vi "Scan Engine-Single Frame.vi"(8 "Error in":errorcluster, 10 "Scan Status in":T1) -> (0 "Error Out":errorcluster, 2 "Buffer":u16[](array[numeric]), 3 "FFT Buffer":sgl[](array[numeric]))   [LabVIEW 2018]
uses:
  Controls/scan status.ctl
  Controls/FGV Actions.ctl
  Hardware Mfg/AlazarTech SDK/Controls/Alazar Engine Actions.ctl
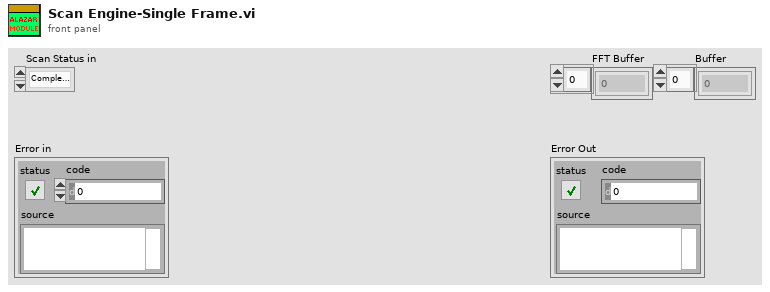
[diagram p1: front panel]
types:
  T1 = typedef "scan status.ctl" = enum16{"Complete Scan(ThorOCT)", "Complete Scan(PSOCT)", "Start(ThorOCT Spatial)", "Start(ThorOCT Spectral)", "Start(GPU FFT)", "Start(Alazar FFT)", "Scan(ThorOCT Spatial)", "Scan(ThorOCT Spectral)", "Scan(GPU FFT)", "Scan(Alazar FFT)", "Finish Scan(ThorOCT)", "Finish Scan(PSOCT)", "Scan(simulate)", "Start(ROI)"}
  T2 = typedef "FGV Actions.ctl" = enum16{"Init", "Set", "Get", "Clear"}
  T3 = typedef "System Parameters.ctl" = cluster{"Optical Parameters":T4, "Vibratome":T5, "Table Stages":T7, "Imaging Parameter":T10, "Galvo HW Parameters":cluster{"Analog Out Channel":tag, "Min Voltage":dbl, "Max Voltage":dbl, "Pixel Clock Source":tag, "Sample Rate":dbl, "Line Clock Out Ch":tag, "2P ready check":tag}, "Alazar parameters":T12, "Mosaic Paramter":cluster{"X Axis":cluster{"Start [mm]":dbl, "Steps [pts]":dbl, "End [mm]":dbl}, "Y Axis":cluster{"Start [mm]":dbl, "Steps [pts]":dbl, "End [mm]":dbl}, "Scan Pattern":enum16{"Uni-directional", "Bi-Directional", "Spiral Out", "Spiral In"}, "Overlap Options":cluster{"Overlap Type":enum16{"No Overlap", "X Only", "Y Only", "X and Y"}, "Percent Overlap":u8, "Justify":enum16{"Start", "Center", "End"}}}, "Manual Controls":T19, "Z stage setting":T23, "Attenuator":T24}
  T4 = typedef "Optical Parameters.ctl" = cluster{"Obj. Focal Length [mm]":dbl, "Scan Lens EFL[mm]":dbl, "Tube Lens EFL[mm]":dbl, "Galvo V Range (+/-)":dbl, "Galvo Max Half Angle [Deg]":dbl, "Max Galvo Range[%]":dbl}
  T5 = typedef "Vibratome Parameters.ctl" = cluster{"Pre Cut Dwell [s]":dbl, "Blade Frequency [RPM]":u16, "Slice Speed [mm/s]":dbl, "Post Cut Dwell [s]":dbl, "Ramp Time [s]":dbl, "Start X [mm]":dbl, "Start Y [mm]":dbl, "Slice Length [mm]":dbl, "Slice Axis":enum16{"X Axis", "Y Axis", "Z Axis"}, "Controller VISA Ref":refnum<visa-resource-name>, "Blade Frequency [Hz]":u16, "Analog Out Channel":tag, "Pixel Clock Source":tag, "Vib version":T6}
  T6 = typedef "vibratome.ctl" = enum16{"Vibratome1", "Vibratome3"}
  T7 = typedef "Translation Stage Parameters.ctl" = cluster{"X Stage":T8, "Y Stage":T8, "Z Stage":T8, "Attenuator":T8}
  T8 = typedef "Translation Stage Cluster.ctl" = cluster{"Position":dbl, "Is.Enabled?":bool, "Is.Connected?":bool, "Device SN":string, "AccelerationMaximum":dbl, "VelocityMaximum":dbl, "Acceleration":dbl, "Velocity":dbl, "waitTimeout (ms)":i32, "Model":T9, "Is.Homed?":bool, "MOVE":bool}
  T9 = typedef "Translation Stage Types.ctl" = enum16{"None", "Thorlabs LTS", "Thorlabs MLJ"}
  T10 = typedef "Imaging Parameters.ctl" = cluster{"Raster Scan Direction":T11, "Pixel Dwell Time [Clock Cycles]":u16, "Flyback Time [Clock Cycles]":u16, "XY Center [um]":cluster{"X":dbl, "Y":dbl}, "Pixel Step Size [um] X":dbl, "XY Image Size":enum16{"32 x 32", "64 x 64", "128 x 128", "256 x 256", "512 x 512", "1024 x 1024", "2048 x 2048"}, "Custom":bool, "Custom Size":cluster{"X":u16, "Y":u16}, "Line Averages":u16, "Pixel Step Size [um] Y":dbl}
  T11 = typedef "Scan Direction.ctl" = enum16{"Uni Directional", "Bi Directional", "None"}
  T12 = typedef "Alazar parameters.ctl" = cluster{"Trigger Settings":cluster{"General Trigger Settings":T13, "Trigger Engine 1":T14, "Trigger Engine 2":T14}, "Device ID":T15, "Ch A Input Control":T16, "Ch B Input Control":T16, "Acq Settings":T17, "Capture Clock":T18}
  T13 = typedef "General Trigger Settings.ctl" = cluster{"Trigger Operation":u32, "Coupling ID":u32, "Range ID":u32, "Delay":u32, "Timeout Ticks":u32, "Mode":u32, "Parameter":u32}
  T14 = typedef "Trigger Engine Controls.ctl" = cluster{"Trigger Engine":u32, "Source":u32, "Slope":u32, "Level":u32}
  T15 = typedef "Alazar Device ID.ctl" = cluster{"System ID":u32, "Board ID":u32}
  T16 = typedef "Channel Input Controls.ctl" = cluster{"Channel":u8, "Coupling":u32, "Range":u32, "Impedance":u32}
  T17 = typedef "Alazar Acquisition Settings.ctl" = cluster{"Record Length":u32, "Offset":u32, "Records Per Buffer":u32, "Records Count (Records/Acq)":u32, "Window Type":u32, "Footer":u32, "Samples per record":u32, "Output Format":u32}
  T18 = typedef "Clock Controls.ctl" = cluster{"Sample Rate":u32, "Decimation":u32, "Source":u32, "Edge":u32}
  T19 = typedef "Manual Controls.ctl" = cluster{"Data Path":path, "Save parameters":T20, "Acquisition mode":T21, "PSOCT Channel":u32, "Save data?":bool, "AIP rotation angle":dbl, "Pause acquisition?":bool, "Outgoing Mail Server (SMTP)":string, "Email":string, "Password":string, "Carrier 1":enum16{"T-Mobile", "AT&T", "Verizon", "Sprint"}, "phone number 1":string, "Subject":string, "Message":string, "Carrier 2":enum16{"T-Mobile", "AT&T", "Verizon", "Sprint"}, "phone number 2":string, "Check boundary?":bool, "Threshold":sgl, "Outputs for GPU FFT":T22, "Slice# init":i32}
  T20 = typedef "FFT parameters.ctl" = cluster{"start pixel":i32, "#pixels to save":i32}
  T21 = typedef "FFT mode.ctl" = enum16{"ThorOCT B line", "ThorOCT Spectral", "ThorOCT FFT", "Alazar B line", "Alazar FFT", "GPU FFT", "Alazar Spectral", "Simulation", "auto adjust focus", "Save all"}
  T22 = typedef "GPU FFT outputs.ctl" = enum16{"Amp + Phase diff", "Amp + Phase", "Amp only"}
  T23 = typedef "Vibratome Param.ctl" = cluster{"first cut height(mm)":dbl, "slice thickness[um]":dbl[], "#repetitions":u16, "image thickness(um)":dbl[], "#cycles per repetition":u16, "First image height(mm)":dbl, "Block?":bool[], "Z0":dbl, "fixed Z0?":bool}
  T24 = typedef "attenuator.ctl" = cluster{"Power after Objective (recalibrate every 6 month)":dbl[]}
  T25 = typedef "Alazar Engine Actions.ctl" = enum16{"Init", "Config Clock", "Config Ch", "Config Trig", "Config Non-FFT Acq.", "Non-FFT Acquire", "start acquire", "Config Acq.", "Acquire", "UnInit"}
  T26 = enum16{"Configure channels", "Write Scan Pattern", "Start Galvo Task", "Is Task Done?", "Stop Galvo", "Uninit", "Init: Calc scan pattern"}
  T27 = cluster{"General Trigger Settings":T13, "Trigger Engine 1":T14, "Trigger Engine 2":T14}
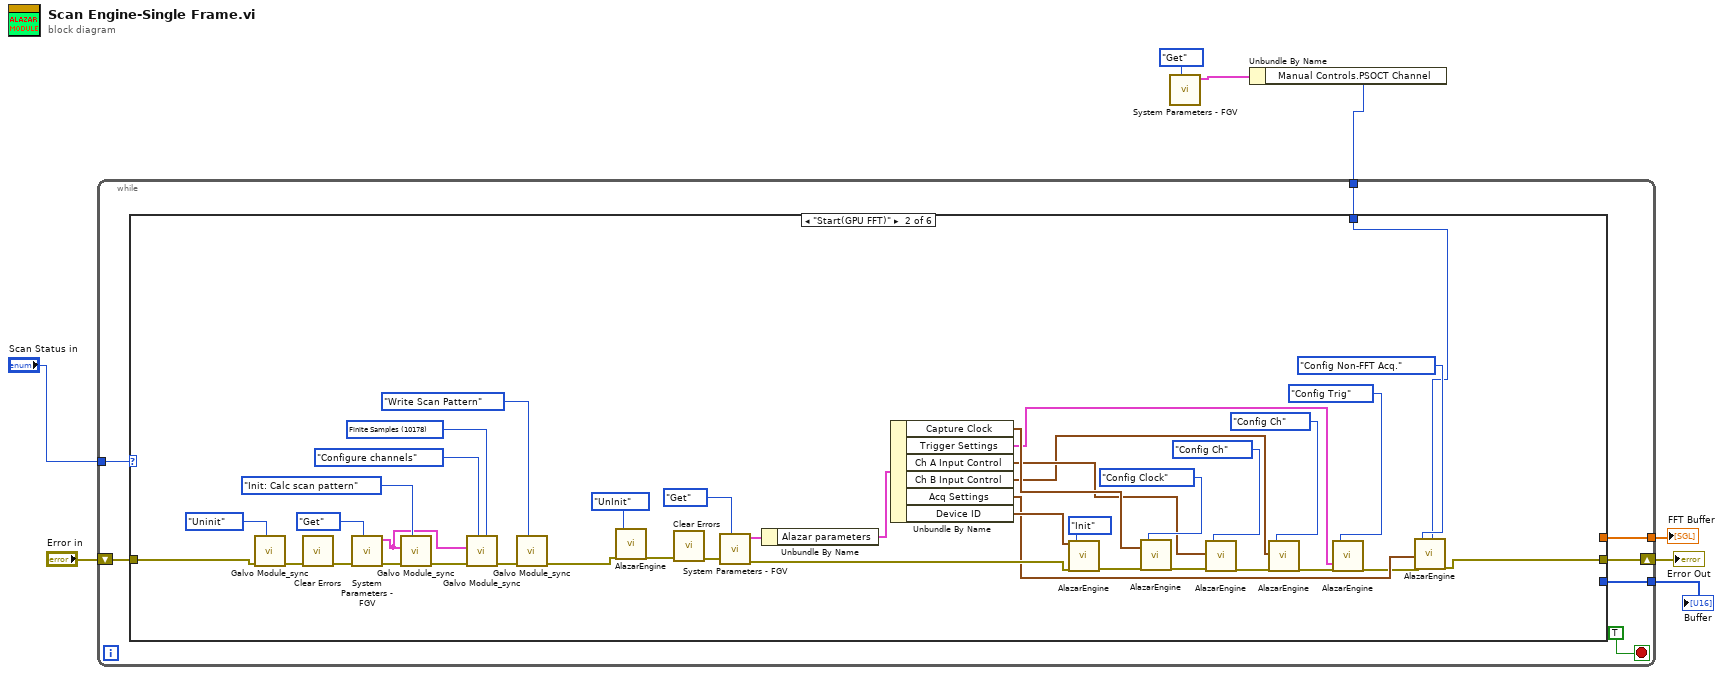
[diagram p0: block diagram]
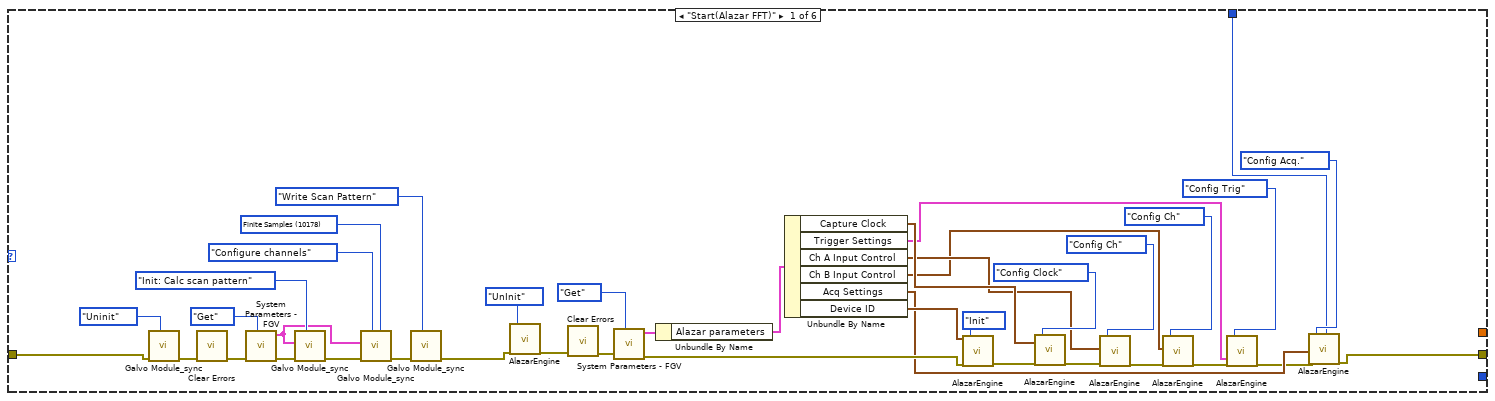
[diagram p2: hidden frame]
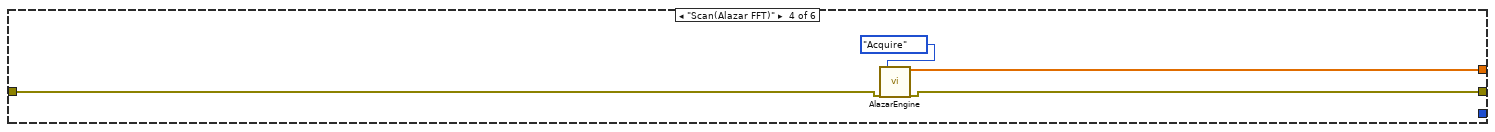
[diagram p4: hidden frame]
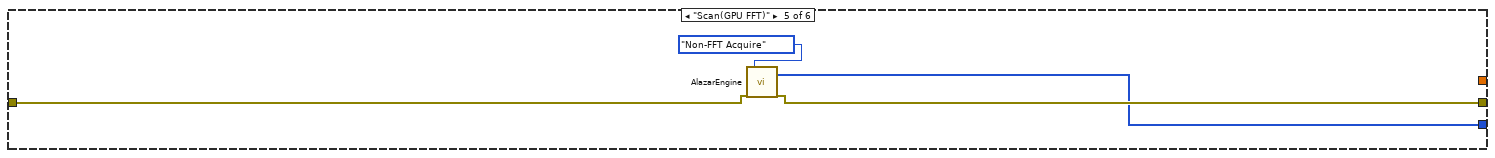
[diagram p5: hidden frame]
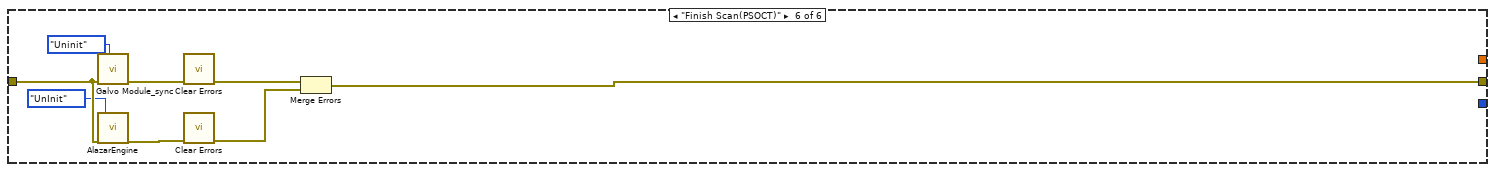
[diagram p6: hidden frame]
diagram:
  n1 = call "System Parameters - FGV.vi"("Actions"=FGV_Actions."Get") -> ("System Parameters [Out]"=w2:T3)  [unwired: 9 in, 1 out]
  n2 = Unbundle By Name(w2) -> ("Manual Controls.PSOCT Channel"=w1:u32)
  n3 = while {
    shift-right: [w14] -> w7
    shift-left: "Error in" -> [w12]
    tunnel: "Scan Status in" -> [w13]
    tunnel: [w11] -> w5
    tunnel: [w10] -> w4
    tunnel: w1 -> [w9]
    stop <- TRUE ("Status In") stop-if-true
    n4 = case shown="\"Start(GPU FFT)\"" w13 {
      tunnel: w12 -> [w44 w59 w96 w99 w103 w109]
      tunnel: [w18 w58 w96 w98 w102 w106] -> w14
      tunnel: [_ _ _ w97 _ _] -> w11
      tunnel: [_ _ _ _ w101 _] -> w10
      tunnel: w9 -> [w17 w57 _ _ _ _]
      frame "Start(Alazar FFT)" {
        w52 = 10178 items=["Finite Samples"=10178, "Continuous Samples"=10123, "Hardware Timed Single Point"=12522] ("sample mode")
        n5 = call "Galvo Module_sync.vi"("Action"=T26."Uninit", "error in (no error)"=w44) -> ("error out"=w47:errorcluster)  [unwired: 8 in, 1 out]
        n6 = call <vilib>:"Clear Errors.vi"("error in (no error)"=w47) -> ("error out"=w45:errorcluster)  [unwired: 5 in, 1 out]
        n7 = call "System Parameters - FGV.vi"("Actions"=FGV_Actions."Get", "Error In"=w45) -> ("Error Out"=w48:errorcluster, "System Parameters [Out]"=w16:T3)  [unwired: 8 in]
        n8 = call "Galvo Module_sync.vi"("Action"=T26."Init: Calc scan pattern", "error in (no error)"=w48, "System Parameters"=w16) -> ("error out"=w54:errorcluster)  [unwired: 7 in, 1 out]
        n9 = call "Galvo Module_sync.vi"("sample mode"=w52, "Action"=T26."Configure channels", "error in (no error)"=w54, "System Parameters"=w16) -> ("error out"=w55:errorcluster)  [unwired: 6 in, 1 out]
        n10 = call "Galvo Module_sync.vi"("Action"=T26."Write Scan Pattern", "error in (no error)"=w55) -> ("error out"=w39:errorcluster)  [unwired: 8 in, 1 out]
        n11 = call "AlazarEngine.vi"("error in (no error)"=w39, "Action"=Alazar_Engine_Actions."UnInit") -> ("error out"=w38:errorcluster)  [unwired: 15 in, 2 out]
        n12 = call <vilib>:"Clear Errors.vi"("error in (no error)"=w38) -> ("error out"=w40:errorcluster)  [unwired: 5 in, 1 out]
        n13 = call "System Parameters - FGV.vi"("Actions"=FGV_Actions."Get", "Error In"=w40) -> ("Error Out"=w30:errorcluster, "System Parameters [Out]"=w42:T3)  [unwired: 8 in]
        n14 = Unbundle By Name(w42) -> ("Alazar parameters"=w41:T12)
        n15 = Unbundle By Name(w41) -> ("Capture Clock"=w28:T18, "Trigger Settings"=w25:T27, "Ch A Input Control"=w27:T16, "Ch B Input Control"=w26:T16, "Acq Settings"=w24:T17, "Device ID"=w29:T15)
        n16 = call "AlazarEngine.vi"("Device ID"=w29, "error in (no error)"=w30, "Action"=Alazar_Engine_Actions."Init") -> ("error out"=w23:errorcluster)  [unwired: 14 in, 2 out]
        n17 = call "AlazarEngine.vi"("Capture Clock"=w28, "error in (no error)"=w23, "Action"=Alazar_Engine_Actions."Config Clock") -> ("error out"=w22:errorcluster)  [unwired: 14 in, 2 out]
        n18 = call "AlazarEngine.vi"("Ch Input Control"=w27, "error in (no error)"=w22, "Action"=Alazar_Engine_Actions."Config Ch") -> ("error out"=w21:errorcluster)  [unwired: 14 in, 2 out]
        n19 = call "AlazarEngine.vi"("Ch Input Control"=w26, "error in (no error)"=w21, "Action"=Alazar_Engine_Actions."Config Ch") -> ("error out"=w20:errorcluster)  [unwired: 14 in, 2 out]
        n20 = call "AlazarEngine.vi"("Trigger Settings"=w25, "error in (no error)"=w20, "Action"=Alazar_Engine_Actions."Config Trig") -> ("error out"=w19:errorcluster)  [unwired: 14 in, 2 out]
        n21 = call "AlazarEngine.vi"("Acq Settings"=w24, "error in (no error)"=w19, "Action"=Alazar_Engine_Actions."Config Acq.", "FFT Channel"=w17) -> ("error out"=w18:errorcluster)  [unwired: 13 in, 2 out]
      }
      frame "Start(GPU FFT)" {
        w92 = 10178 items=["Finite Samples"=10178, "Continuous Samples"=10123, "Hardware Timed Single Point"=12522] ("sample mode")
        n22 = call "Galvo Module_sync.vi"("Action"=T26."Uninit", "error in (no error)"=w59) -> ("error out"=w87:errorcluster)  [unwired: 8 in, 1 out]
        n23 = call <vilib>:"Clear Errors.vi"("error in (no error)"=w87) -> ("error out"=w85:errorcluster)  [unwired: 5 in, 1 out]
        n24 = call "System Parameters - FGV.vi"("Actions"=FGV_Actions."Get", "Error In"=w85) -> ("Error Out"=w88:errorcluster, "System Parameters [Out]"=w56:T3)  [unwired: 8 in]
        n25 = call "Galvo Module_sync.vi"("Action"=T26."Init: Calc scan pattern", "error in (no error)"=w88, "System Parameters"=w56) -> ("error out"=w94:errorcluster)  [unwired: 7 in, 1 out]
        n26 = call "Galvo Module_sync.vi"("sample mode"=w92, "Action"=T26."Configure channels", "error in (no error)"=w94, "System Parameters"=w56) -> ("error out"=w95:errorcluster)  [unwired: 6 in, 1 out]
        n27 = call "Galvo Module_sync.vi"("Action"=T26."Write Scan Pattern", "error in (no error)"=w95) -> ("error out"=w80:errorcluster)  [unwired: 8 in, 1 out]
        n28 = call "AlazarEngine.vi"("error in (no error)"=w80, "Action"=Alazar_Engine_Actions."UnInit") -> ("error out"=w79:errorcluster)  [unwired: 15 in, 2 out]
        n29 = call <vilib>:"Clear Errors.vi"("error in (no error)"=w79) -> ("error out"=w81:errorcluster)  [unwired: 5 in, 1 out]
        n30 = call "System Parameters - FGV.vi"("Actions"=FGV_Actions."Get", "Error In"=w81) -> ("Error Out"=w71:errorcluster, "System Parameters [Out]"=w83:T3)  [unwired: 8 in]
        n31 = Unbundle By Name(w83) -> ("Alazar parameters"=w82:T12)
        n32 = Unbundle By Name(w82) -> ("Capture Clock"=w69:T18, "Trigger Settings"=w66:T27, "Ch A Input Control"=w68:T16, "Ch B Input Control"=w67:T16, "Acq Settings"=w65:T17, "Device ID"=w70:T15)
        n33 = call "AlazarEngine.vi"("Device ID"=w70, "error in (no error)"=w71, "Action"=Alazar_Engine_Actions."Init") -> ("error out"=w64:errorcluster)  [unwired: 14 in, 2 out]
        n34 = call "AlazarEngine.vi"("Capture Clock"=w69, "error in (no error)"=w64, "Action"=Alazar_Engine_Actions."Config Clock") -> ("error out"=w63:errorcluster)  [unwired: 14 in, 2 out]
        n35 = call "AlazarEngine.vi"("Ch Input Control"=w68, "error in (no error)"=w63, "Action"=Alazar_Engine_Actions."Config Ch") -> ("error out"=w62:errorcluster)  [unwired: 14 in, 2 out]
        n36 = call "AlazarEngine.vi"("Ch Input Control"=w67, "error in (no error)"=w62, "Action"=Alazar_Engine_Actions."Config Ch") -> ("error out"=w61:errorcluster)  [unwired: 14 in, 2 out]
        n37 = call "AlazarEngine.vi"("Trigger Settings"=w66, "error in (no error)"=w61, "Action"=Alazar_Engine_Actions."Config Trig") -> ("error out"=w60:errorcluster)  [unwired: 14 in, 2 out]
        n38 = call "AlazarEngine.vi"("Acq Settings"=w65, "error in (no error)"=w60, "Action"=Alazar_Engine_Actions."Config Non-FFT Acq.", "FFT Channel"=w57) -> ("error out"=w58:errorcluster)  [unwired: 13 in, 2 out]
      }
      frame Default {
      }
      frame "Scan(Alazar FFT)" {
        n39 = call "AlazarEngine.vi"("error in (no error)"=w99, "Action"=Alazar_Engine_Actions."Acquire") -> ("FFT Buffer"=w97:sgl[], "error out"=w98:errorcluster)  [unwired: 15 in, 1 out]
      }
      frame "Scan(GPU FFT)" {
        n40 = call "AlazarEngine.vi"("error in (no error)"=w103, "Action"=Alazar_Engine_Actions."Non-FFT Acquire") -> ("Buffer"=w101:u16[], "error out"=w102:errorcluster)  [unwired: 15 in, 1 out]
      }
      frame "Finish Scan(PSOCT)" {
        n41 = call "Galvo Module_sync.vi"("Action"=T26."Uninit", "error in (no error)"=w109) -> ("error out"=w112:errorcluster)  [unwired: 8 in, 1 out]
        n42 = call "AlazarEngine.vi"("error in (no error)"=w109, "Action"=Alazar_Engine_Actions."UnInit") -> ("error out"=w111:errorcluster)  [unwired: 15 in, 2 out]
        n43 = call <vilib>:"Clear Errors.vi"("error in (no error)"=w112) -> ("error out"=w108:errorcluster)  [unwired: 5 in, 1 out]
        n44 = call <vilib>:"Clear Errors.vi"("error in (no error)"=w111) -> ("error out"=w107:errorcluster)  [unwired: 5 in, 1 out]
        n45 = Merge Errors(w108, w107) -> (w106:errorcluster)
      }
    }
  }
  "Error Out" <- w7
  "FFT Buffer" <- w5
  "Buffer" <- w4
